vi "Upload File to Bucket.vi"() -> ()   [LabVIEW 2015]
doc: "Demonstrates how to upload a file from the local file system to an Amazon S3 bucket."
uses:
  Typedefs/AMZ_S3_LocationConstraint.ctl
  Typedefs/AMZ_S3_AWS Credentials.ctl
  Typedefs/AMZ_S3_ACL.ctl
  Typedefs/AMZ_S3_API_PUT Object Request Parameters.ctl
  Typedefs/AMZ_S3_Storage Class.ctl
  Typedefs/AMZ_S3_Object Metadata.ctl
  Typedefs/AMZ_S3_API_POST Multipart Object Request Parameters.ctl
  LV Interface for Amazon S3.lvlib
panel:
  in  "Region":T1
  in  "File to Upload":path
  in  "Secret Key":string
  in  "Access Key":string
  out "New Object Location":string
  in  "Public":bool
  in  "Object Path":string="uploads/"
  in  "Destination Bucket":string
  # "Overview: Demonstrates how to upload a file to an Amazon S3 bucket.\nRequirements: LabVIEW Interface for Amazon S3 toolkit and a registered Amazon AWS account\nInstructions:\n1. Specify the Access Key and Secret Key for your AWS account. You can create an account at http://aws.amazon.com.\n2. Specify a Destination Bucket for the file. If you have not created a bucket, you can run the Create a new bucket.vi example to create a new bucket.\n3. Set Public to TRUE if you want the file to be public.\n4. Specify the Region the bucket is located in.\n5. Specify the File to Upload.\n6. Set the Object Path if you want to store the file in a folder within the bucket.\n7. Run the VI. Observe the URL of the stored file in the New Object Location indicator."
  # "Note: If you set Public to FALSE, you will not be able to download the file using the New Object Location URL. This is because you must use an authentication method to access non-public objects."
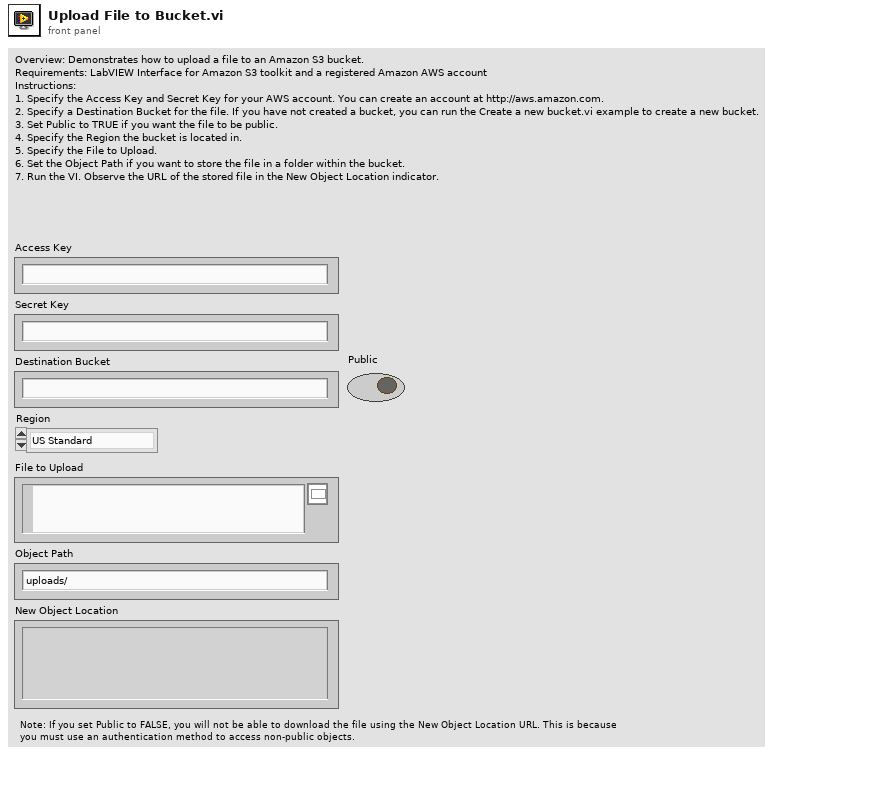
[diagram p1: front panel]
types:
  T1 = typedef "LV Interface for Amazon S3.lvlib/AMZ_S3_LocationConstraint.ctl" = enum16{"US Standard", "us-east-2", "us-west-1", "us-west-2", "ap-northeast-1", "ap-northeast-2", "ap-southeast-1", "ap-southeast-2", "ca-central-1", "eu-central-1", "eu-west-1", "eu-west-2", "sa-east-1"}
  T2 = typedef "LV Interface for Amazon S3.lvlib/AMZ_S3_AWS Credentials.ctl" = cluster{"Access Key":string, "Secret Key":string}
  T3 = typedef "LV Interface for Amazon S3.lvlib/AMZ_S3_ACL.ctl" = enum16{"private", "public-read", "public-read-write", "aws-exec-read", "authenticated-read", "bucket-owner-read", "bucket-owner-full-control"}
  T4 = typedef "LV Interface for Amazon S3.lvlib/AMZ_S3_API_PUT Object Request Parameters.ctl" = cluster{"Content Type":string, "ACL":T3, "Storage Class":T5, "User Metadata":T6[], "Content MD5":string}
  T5 = typedef "LV Interface for Amazon S3.lvlib/AMZ_S3_Storage Class.ctl" = enum16{"STANDARD", "REDUCED_REDUNDANCY"}
  T6 = typedef "LV Interface for Amazon S3.lvlib/AMZ_S3_Object Metadata.ctl" = cluster{"Key":string, "Value":string}
  T7 = typedef "LV Interface for Amazon S3.lvlib/AMZ_S3_API_POST Multipart Object Request Parameters.ctl" = cluster{"Content Type":string, "ACL":T3, "Storage Class":T5, "User Metadata":T6[]}
  T8 = typedef "LV Interface for Amazon S3.lvlib/AMZ_S3_API_CompleteMultipartUploadResult.ctl" = cluster{"Location":string, "Bucket":string, "Key":string, "ETag":string}
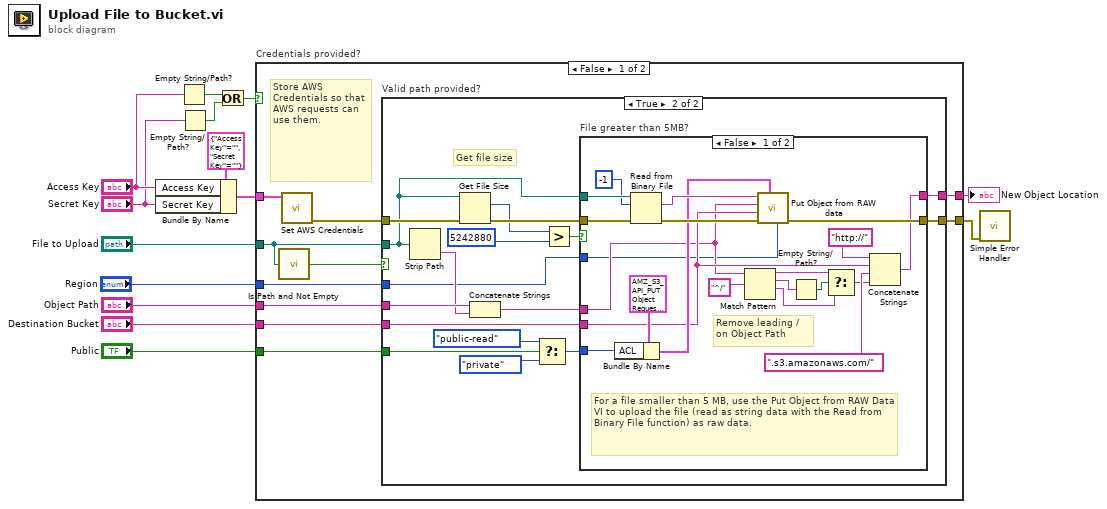
[diagram p0: block diagram]
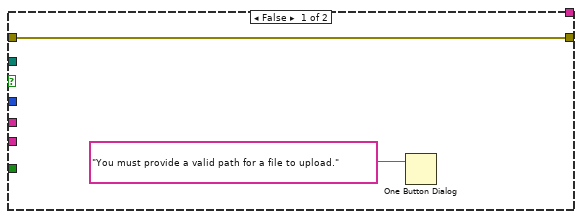
[diagram p2: hidden frame]
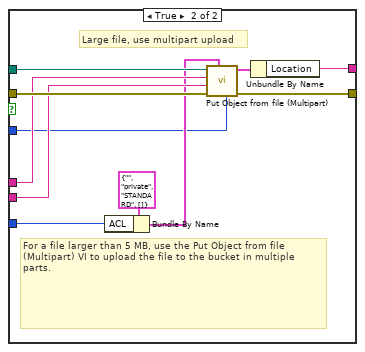
[diagram p3: hidden frame]
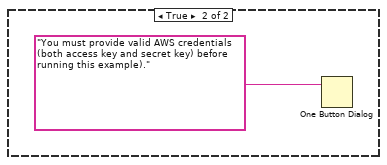
[diagram p4: hidden frame]
diagram:
  n1 = Bundle By Name(cluster=T2 {"Access Key"="", "Secret Key"=""} ("AWS Credentials in"), "Access Key"="Access Key", "Secret Key"="Secret Key") -> (w7:T2)
  n2 = Empty String/Path?(string/path="Access Key") -> (empty?=w12:bool)
  n3 = Empty String/Path?(string/path="Secret Key") -> (empty?=w13:bool)
  n4 = Or(x=w12, y=w13) -> (x .or. y?=w8:bool)
  n5 = case "Credentials provided?" shown="False" w8 {
    tunnel: w7 -> [w24 _]
    tunnel: [w23 _] -> w14
    tunnel: "File to Upload" -> [w21 _]
    tunnel: "Destination Bucket" -> [w19 _]
    tunnel: "Public" -> [w18 _]
    tunnel: "Object Path" -> [w17 _]
    tunnel: "Region" -> [w16 _]
    tunnel: [w15 _] -> w1
    frame False {
      # "Store AWS Credentials so that AWS requests can use them."
      n6 = call <vilib>:"Is Path and Not Empty.vi"("path"=w21) -> ("Is Path and Not Empty?"=w20:bool)  [unwired: 4 in]
      n7 = call "Set AWS Credentials.vi"("AWS Credentials in"=w24) -> ("error out"=w22:errorcluster)  [unwired: 10 in]
      n8 = case "Valid path provided?" shown="True" w20 {
        tunnel: w22 -> [w25 w42]
        tunnel: w21 -> [_ w29]
        tunnel: [_ w43] -> w23
        tunnel: w19 -> [_ w34]
        tunnel: w18 -> [_ w33]
        tunnel: w17 -> [_ w32]
        tunnel: w16 -> [_ w28]
        tunnel: [w25 w27] -> w15
        frame False {
          n9 = One Button Dialog(message="You must provide a valid path for a file to upload.") -> ()  [unwired: 1 in, 1 out]
        }
        frame True {
          # "Get file size"
          n10 = Strip Path(path=w29) -> (name=w30:string)  [unwired: 1 out]
          n11 = Get File Size(file=w29, error in=w42) -> (size (in bytes)=w40:i64, 0:w41:errorcluster)  [unwired: 1 out]
          n12 = Concatenate Strings(w32, w30) -> (w31:string)
          n13 = Select(t=AMZ_S3_ACL."public-read" ("ACL"), s=w33, f=AMZ_S3_ACL."private" ("ACL")) -> (s? t:f=w35:T3)
          n14 = Greater?(x=w40, y=i64 5242880) -> (0:w38:bool)
          n15 = case "File greater than 5MB?" shown="False" w38 {
            tunnel: w41 -> [w64 w75]
            tunnel: w29 -> [w63 w74]
            tunnel: w34 -> [w53 w72]
            tunnel: w31 -> [w45 w73]
            tunnel: w35 -> [w58 w67]
            tunnel: [w56 w71] -> w27
            tunnel: [w52 w69] -> w43
            tunnel: w28 -> [w44 w65]
            frame False {
              # "Remove leading / \non Object Path"
              # "For a file smaller than 5 MB, use the Put Object from RAW Data VI to upload the file (read as string data with the Read from Binary File function) as raw data."
              n16 = Bundle By Name(cluster=T4 {"Content Type"="", "ACL"=enum."private", "Storage Class"=enum."STANDARD", "User Metadata"=[], "Content MD5"=""} ("Request Parameters"), "ACL"=w58) -> (w57:T4)
              n17 = Read from Binary File(8:w64, 10:-1 ("count (1)"), 11:w63) -> (0:w61:errorcluster, 2:w60:string)  [unwired: 3 in, 2 out]
              n18 = Match Pattern(string=w45, regular expression="^/") -> (before substring=w50:string, match substring=w48:string, after substring=w51:string)  [unwired: 1 in, 1 out]
              n19 = call "Put Object from RAW data.vi"("Region"=w44, "Request Parameters"=w57, "error in (no error)"=w61, "Bucket"=w53, "Object Path"=w45, "Data"=w60) -> ("error out"=w56:errorcluster)  [unwired: 4 in, 1 out]
              n20 = Empty String/Path?(string/path=w48) -> (empty?=w49:bool)
              n21 = Select(t=w50, s=w49, f=w51) -> (s? t:f=w46:string)
              n22 = Concatenate Strings("http://" ("string"), w53, ".s3.amazonaws.com/" ("string"), w46) -> (w52:string)
            }
            frame True {
              # "For a file larger than 5 MB, use the Put Object from file (Multipart) VI to upload the file to the bucket in multiple parts."
              # "Large file, use multipart upload"
              n23 = Bundle By Name(cluster=T7 {"Content Type"="", "ACL"=enum."private", "Storage Class"=enum."STANDARD", "User Metadata"=[]} ("Request Parameters"), "ACL"=w67) -> (w66:T7)
              n24 = call "Put Object from file (Multipart).vi"("Region"=w65, "Request Parameters"=w66, "error in (no error)"=w75, "Bucket"=w72, "Object Path"=w73, "Local file path"=w74) -> ("error out"=w71:errorcluster, "CompleteMultipartUploadResult"=w70:T8)  [unwired: 3 in, 1 out]
              n25 = Unbundle By Name(w70) -> ("Location"=w69:string)
            }
          }
        }
      }
    }
    frame True {
      n26 = One Button Dialog(message="You must provide valid AWS credentials (both access key and secret key) before running this example).") -> ()  [unwired: 1 in, 1 out]
    }
  }
  "New Object Location" <- w14
  n27 = call <vilib>:"Simple Error Handler.vi"("error in (no error)"=w1) -> ()  [unwired: 4 in, 5 out]
